vi "SetCurrentPathIndex.vi"(8 "error in (no error)":errorcluster, 11 "Setting Database in":refnum<class "Setting Database.lvclass">) -> (0 "error out":errorcluster, 3 "Setting Database out":refnum<class "Setting Database.lvclass">)   [LabVIEW 2020, in "Setting Database.lvclass"]
uses:
  Setting Database.lvclass
panel:
  in  "Index":i32
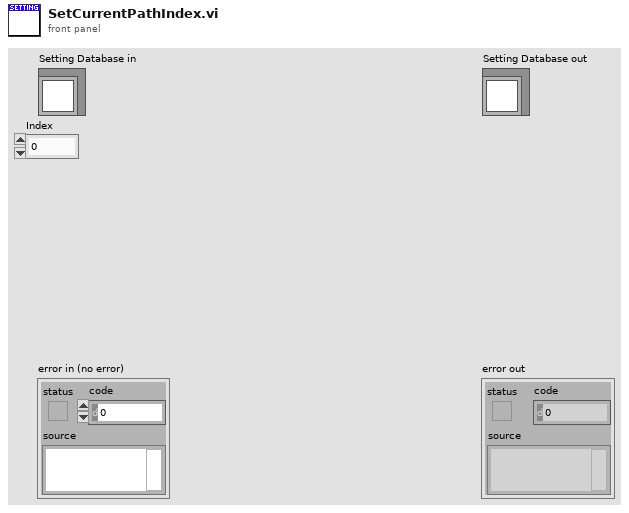
[diagram p1: front panel]
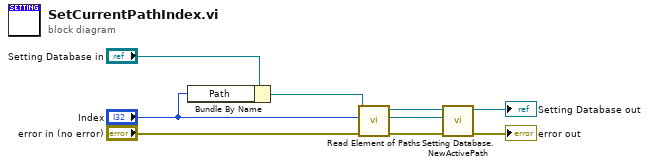
[diagram p0: block diagram]
diagram:
  n1 = Bundle By Name(cluster="Setting Database in", "Path"="Index") -> (w2:refnum<class "Setting Database.lvclass">)
  n2 = call "Read Element of Paths.vi"("error in (no error)"="error in (no error)", 10:"Index", "Setting Database in"=w2) -> ("error out"=w6:errorcluster, "Path Settings.lvclass"=w7:refnum<class "Path Settings.lvclass">, "Setting Database out"=w4:refnum<class "Setting Database.lvclass">)  [unwired: 6 in]
  n3 = call "Setting Database.NewActivePath.vi"("error in (no error)"=w6, "NewCurrentPath"=w7, "Setting Database"=w4) -> ("error out"=→"error out":errorcluster, "Setting Database"=→"Setting Database out":refnum<class "Setting Database.lvclass">)  [unwired: 7 in]
